vi "ILABR_CreateFromTemplate.vi"(0 "path":string, 3 "port":i32, 4 "machineName":string, 5 "suffix":string, 6 "templateName":string) -> (1 "viReference":refnum<vi>, 2 "name":string)   [LabVIEW 2009]
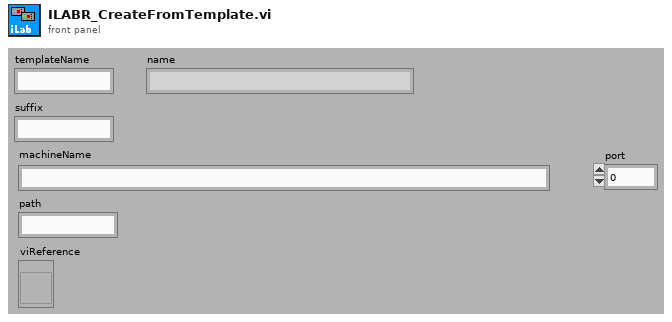
[diagram p1: front panel]
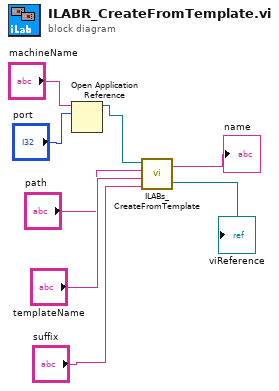
[diagram p0: block diagram]
diagram:
  n1 = Open Application Reference(10:"port", 11:"machineName") -> (3:w6:refnum<vi>)  [unwired: 1 in, 2 out]
  n2 = call "ILABs_CreateFromTemplate.vi"("suffix"="suffix", "templateName"="templateName", "path"="path", "appRef"=w6) -> ("viReference"=→"viReference":refnum<vi>, "name"=→"name":string)
